vi "Input Multiplexer to FFT (2 inputs).vi"(7 "Reset?":bool, 8 "Input Data Valid Array":bool[](array[boolean])=[FALSE, FALSE], 11 "Input Data":T1[](array[typedef])=[0.0, 0.0]) -> (0 "Output Data Valid Array":bool[](array[boolean]), 3 "Interchanged Data":T1[](array[typedef]) format="%.18g")   [LabVIEW 2011]
uses:
  Interpolation Block/Controls/Interpolation Output Data.ctl
  Input Index(Type) 2 inputs.ctl
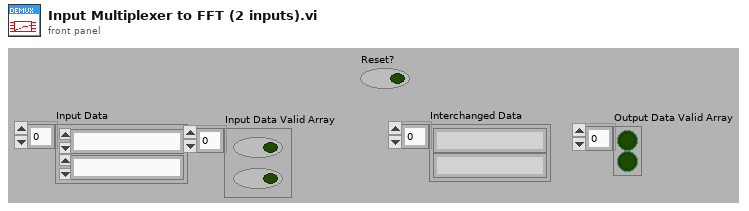
[diagram p1: front panel]
types:
  T1 = typedef "Interpolation Output Data.ctl" = fxp<+/-,19,1>
  T2 = typedef "Input Index(Type) 2 inputs.ctl" = fxp<+,1,1>
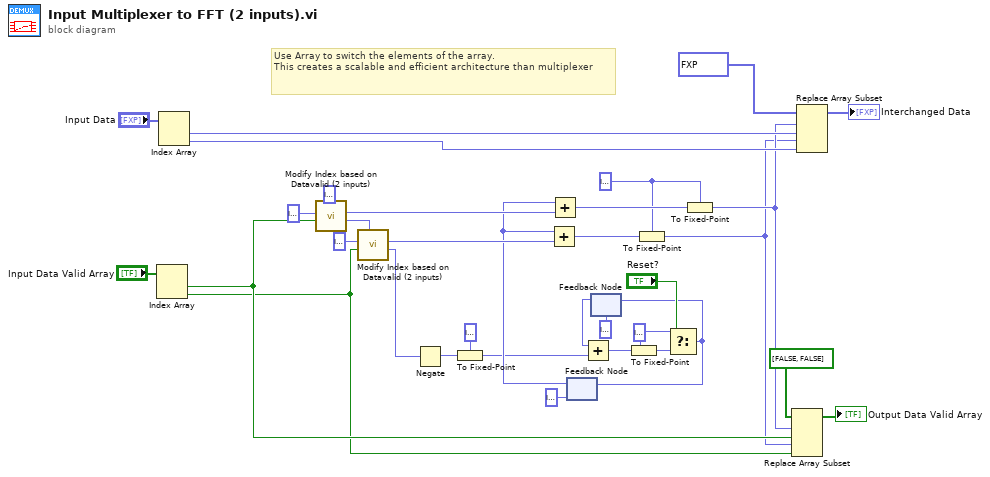
[diagram p0: block diagram]
diagram:
  w13 = T2 0.0
  w5 = T2 0.0 ("Actual Index")
  # "Use Array to switch the elements of the array. \nThis creates a scalable and efficient architecture than multiplexer"
  n1 = Index Array(array="Input Data Valid Array") -> (element #1=w30:bool, element #2=w29:bool)  [unwired: 2 in]
  n2 = Index Array(array="Input Data") -> (element #1=w21:T1, element #2=w20:T1)  [unwired: 2 in]
  n3 = call "Modify Index based on Datavalid (2 inputs).vi"("previous counter val"=T2 0.0, "cuurent index data valid?"=w30, "Actual Index"=T2 0.0) -> ("Next Counter Val"=w31:T2, "Modified Index"=w28:T2)  [unwired: 7 in]
  n4 = call "Modify Index based on Datavalid (2 inputs).vi"("previous counter val"=w31, "cuurent index data valid?"=w29, "Actual Index"=T2 1.0) -> ("Next Counter Val"=w1:T2, "Modified Index"=w26:T2)  [unwired: 7 in]
  n5 = Negate(x=w1) -> (-x=w9:fxp<+/-,1,1>)
  n6 = To Fixed-Point(fixed-point type=T2 0.0 ("Current Index Sum"), number=w9) -> (fixed-point=w8:T2)
  n7 = feedback #1(T2 0.0 ("Current Index Sum")) -> (w24:T2)
  n8 = Add(x=w24, y=w26) -> (x+y=w15:fxp<+,2,2>)
  n9 = Add(x=w24, y=w28) -> (x+y=w27:fxp<+,2,2>)
  n10 = feedback #2(T2 0.0) -> (w23:T2)
  n11 = Add(x=w23, y=w8) -> (x+y=w14:fxp<+,2,2>)
  n12 = To Fixed-Point(fixed-point type=w5, number=w14) -> (fixed-point=w6:T2)
  n13 = To Fixed-Point(fixed-point type=w13, number=w15) -> (fixed-point=w10:T2)
  n14 = Select(t=w5, s="Reset?", f=w6) -> (s? t:f=w3:T2)
  n15 = feedback-in #1(w3) -> ()
  n16 = feedback-in #2(w3) -> ()
  n17 = To Fixed-Point(fixed-point type=w13, number=w27) -> (fixed-point=w11:T2)
  n18 = Replace Array Subset(array=bool[] [FALSE, FALSE] ("appended array"), new element #1=w30, index #1=w11, new element #2=w29, index #2=w10) -> (→"Output Data Valid Array":bool[])
  n19 = Replace Array Subset(array=T1[] [0.0, 0.0], new element #1=w21, index #1=w11, new element #2=w20, index #2=w10) -> (→"Interchanged Data":T1[])
